vi "NI6071E.constructor.vi"(0 "name":string, 2 "data in":string, 5 "error in":errorcluster) -> (14 "i ref out":refnum<vi>, 16 "data out":string, 19 "error out":errorcluster)   [LabVIEW 2014, in "NI6071E.lvlib"]
doc: "This class is forseen to measure the current of the pulsed power of PHELIX. It interacts with a DAQ card in an NI PXI Chasis.\n\nThis class is part of the PHELIX device layer.\n\nauthor: Holger Brand, GSI\n\nLicense Agreement for this software:\n\nCopyright (C)\nGesellschaft für Schwerionenforschung, GSI\nPlanckstr. 1\n64291 Darmstadt\nGermany\n\nContact: D.Beck@gsi.de \n\nThis program is free software; you can redistribute it and/or modify it under the terms of the \nGNU General Public License as published by the Free Software Foundation; either version 2 of \nthe license, or (at your option) any later version.\n\nThis program is distributed in the hope that it will be useful, but WITHOUT ANY WARRANTY; \nwithout even the implied warranty of MERCHANTABILITY or FITNESS FOR A PARTICULAR PURPOSE. See the GNU General License for more details (http://www.gnu.org).\n\nGesellschaft für Schwerionenforschung, GSI\nPlanckstr. 1, 64291 Darmstadt, Germany\nFor all questions and ideas contact: M.Richter@gsi.de, H.Brand@gsi.de or D.Beck@gsi.de.\nLast update: 16-JUN-2004"
uses:
  NI6071E.lvlib
  CSCore/BaseProcess/BaseProcess.lvlib
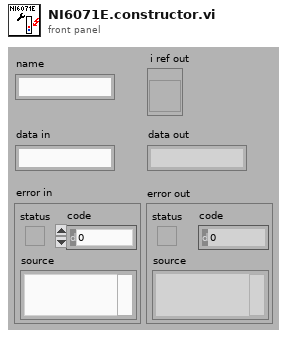
[diagram p1: front panel]
types:
  T1 = enum16{"SetAttribute", "GetAttribute", "CreateAttribute", "DestroyAttribute", "DestroyAllAtributes"}
  T2 = typedef "NI6071E.lvlib/NI6071E.i attribute.ctl" = cluster{"NI6071E Server":string, "Port":u16, "NI6071E Config":T3, "NI6071E Start":T4, "Waveforms":waveform(dbl)[], "RT Error":errorcluster, "NI6071E Read":T5, "connection ID":refnum<k5>, "DAQ Status":string, "device (1)":i16, "DAQ Status Service ID":i32}
  T3 = typedef "NI6071E.lvlib/NI6071EConfig.ctl" = cluster{"device (1)":i16, "channels (0)":tag[], "buffer size (1000 scans)":i32, "[number of buffers] (1)":i32, "measurement mode structure":cluster{"measurement mode":u16, "reserved":u32}, "input limits (no change)":cluster{"high limit (0.0)":sgl, "low limit (0.0)":sgl}[], "coupling & input config (no change:0)":cluster{"coupling (no change:0)":enum16{"no change", "DC", "AC", "GND", "internal ref."}, "input config (no change:0)":u16}[]}
  T4 = typedef "NI6071E.lvlib/NI6071EStart.ctl" = cluster{"scan rate (40000 scans/sec)":sgl, "trigger type (analog)":enum16{"no trigger", "analog", "digital A", "digital A & B", "scan clock gate"}, "edge or slope \n(rising)":enum16{"no change", "rising", "falling"}, "number of buffers to acquire (1)":i32, "analog chan (PFI0) & level (2.00)":cluster{"trigger channel (empty)":string, "level (0.0)":sgl}, "[additional trig params]":cluster{"hysteresis (0.0)":sgl, "coupling (no change:0)":enum16{"no change", "DC", "AC"}, "delay (0 sec)":sgl, "skip count (0)":i32, "time limit (0 sec)":sgl}}
  T5 = typedef "NI6071E.lvlib/NI6071ERead.ctl" = cluster{"time limit in sec (-1:auto calculate)":sgl, "number of scans to read (-1:all)":i32}
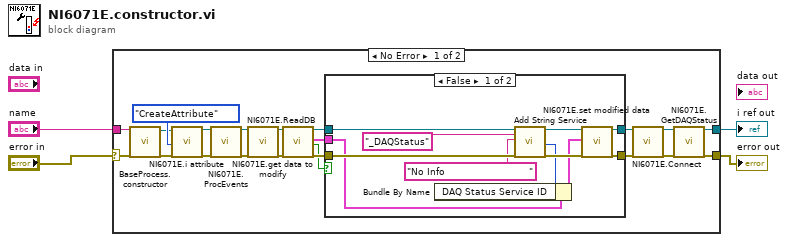
[diagram p0: block diagram]
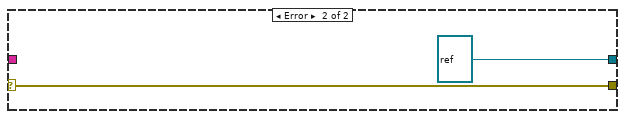
[diagram p3: hidden frame]
diagram:
  n1 = case shown="No Error" "error in" {
    selector: "error in" -> [w17 w40]
    tunnel: "name" -> [w25 _]
    tunnel: [w12 refnum<vi> refnum ("i ref out")] -> w3
    tunnel: [w11 w40] -> w2
    frame No Error {
      n2 = call "BaseProcess.constructor.vi"("name"=w25, "error in (no error)"=w17) -> ("i ref out"=w21:refnum<vi>, "error out"=w20:errorcluster)  [unwired: 15 in, 1 out]
      n3 = call "NI6071E.i attribute.vi"("VI Refnum"=w21, "Action"=T1."CreateAttribute", "error in (no error)"=w20) -> ("VI Refnum out"=w23:refnum<vi>, "error out"=w22:errorcluster)  [unwired: 14 in, 1 out]
      n4 = call "NI6071E.ProcEvents.vi"("i ref in"=w23, "error in"=w22) -> ("i ref out"=w18:refnum<vi>, "error out"=w19:errorcluster)  [unwired: 16 in]
      n5 = call "NI6071E.ReadDB.vi"("i ref in"=w18, "error in"=w19) -> ("i ref out"=w10:refnum<vi>, "error out"=w9:errorcluster)  [unwired: 16 in]
      n6 = call "NI6071E.get data to modify.vi"("i ref in"=w10, "error in (no error)"=w9) -> ("i ref out"=w15:refnum<vi>, "i attribute"=w14:T2, "timed out"=w13:bool, "error out"=w16:errorcluster)  [unwired: 14 in]
      n7 = case shown="False" w13 {
        tunnel: w16 -> [w36 w38]
        tunnel: [w34 w37] -> w5
        tunnel: [w32 w38] -> w7
        tunnel: w15 -> [w31 w37]
        tunnel: w14 -> [w30 _]
        frame False {
          n8 = call "Add String Service.vi"("i ref in"=w31, "Service Name"="_DAQStatus" ("string"), "String"="No Info                            ", "error in (no error)"=w36) -> ("i ref out"=w35:refnum<vi>, "Service ID"=w28:i32, "error out"=w33:errorcluster)  [unwired: 13 in]
          n9 = Bundle By Name(cluster=w30, "DAQ Status Service ID"=w28) -> (w29:T2)
          n10 = call "NI6071E.set modified data.vi"("i ref in"=w35, "i attribute"=w29, "error in (no error)"=w33) -> ("i ref out"=w34:refnum<vi>, "error out"=w32:errorcluster)  [unwired: 15 in]
        }
        frame True {
        }
      }
      n11 = call "NI6071E.Connect.vi"("i ref in"=w5, "error in (no error)"=w7) -> ("i ref out"=w6:refnum<vi>, "error out"=w8:errorcluster)  [unwired: 16 in]
      n12 = call "NI6071E.GetDAQStatus.vi"("i ref in"=w6, "error in (no error)"=w8) -> ("i ref out"=w12:refnum<vi>, "error out"=w11:errorcluster)  [unwired: 15 in, 1 out]
    }
    frame Error {
    }
  }
  "i ref out" <- w3
  "error out" <- w2
